vi "MessageBase.getMessageLength.vi"(8 "error in (no error)":errorcluster, 11 "MessageBase in":refnum<class "MessageBase.lvclass">) -> (0 "error out":errorcluster, 2 "Length":u8, 3 "MessageBase out":refnum<class "MessageBase.lvclass">)   [LabVIEW 2022 SP3, in "MessageBase.lvclass"]
uses:
  MessageBase.lvclass
  MessageBase.lvclass/MessageBase.ctl
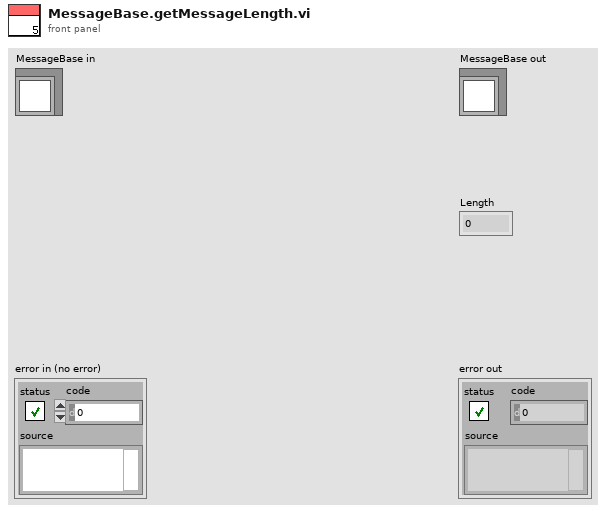
[diagram p1: front panel]
types:
  T1 = typedef "FieldSpec.ctl" = cluster{"Name":string, "Offset":i32, "Length":i32, "FieldType":enum16{"Alphanumeric", "Binary", "BinaryLongPrice", "BinaryShortPrice", "BitField", "PrintableAscii", "Value"}, "FieldValue":variant}
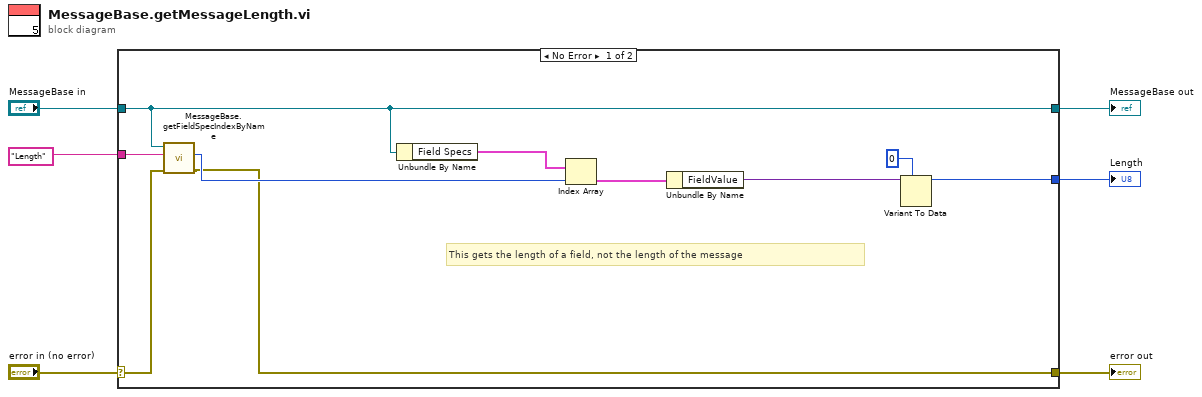
[diagram p0: block diagram]
diagram:
  n1 = case shown="No Error" "error in (no error)" {
    selector: "error in (no error)" -> [w13 w17]
    tunnel: [w12 w17] -> w5
    tunnel: [w11 w18] -> w3
    tunnel: "MessageBase in" -> [w11 w18]
    tunnel: "Length" ("FIeld.Name") -> [w16 _]
    tunnel: [w7 _] -> w1
    frame No Error {
      # "This gets the length of a field, not the length of the message"
      n2 = call-dynamic "MessageBase.getFieldSpecIndexByName.vi"("error in (no error)"=w13, "Field.Name"=w16, "MessageBase in"=w11) -> ("error out"=w12:errorcluster, "Index"=w14:i32)  [unwired: 6 in, 1 out]
      n3 = Unbundle By Name(w11) -> ("Field Specs"=w15:T1[])
      n4 = Index Array(array=w15, index=w14) -> (element=w10:T1)
      n5 = Unbundle By Name(w10) -> ("FieldValue"=w9:variant)
      n6 = Variant To Data(type=u8 0, Variant=w9) -> (data=w7:u8)  [unwired: 1 in, 1 out]
    }
    frame Error {
      # "Wire the error cluster across even in the \"No Error\"\ncase so that warnings get propagated."
    }
  }
  "error out" <- w5
  "MessageBase out" <- w3
  "Length" <- w1
